vi "Path_Test_2020_TankRobot_Ramsete_ScanIndex_CreateFile.vi"() -> ()   [LabVIEW 2019]
uses:
  Pathfinder-Lib/VIs/Waypoint.ctl
  <vilib>/Rock Robotics/WPI/DriverStation/WPI_DriverStationRobotMode2.ctl
  Pathfinder-Lib/VIs/Wheel_Ctrl_Path_Element.ctl
  PathExecution_Library/PATH_SAMPLE.ctl
  PathExecution_Library/POSE.ctl
  PathExecution_Library/TRANSLATION.ctl
  PathExecution_Library/ROTATION.ctl
  Pathfinder-Lib/VIs/Wheel_Ctrl_Path.ctl
  <vilib>/Rock Robotics/SystemInterfaces/AI/FPGA_AIGyroChannel.ctl
  <vilib>/Rock Robotics/SystemInterfaces/DIO/FPGA_DIOChannel.ctl
  <vilib>/Rock Robotics/WPI/Encoder/WPI_EncoderType.ctl
  <vilib>/Rock Robotics/SystemInterfaces/DIO/FPGA_DIOPWMChannel.ctl
  <vilib>/Rock Robotics/WPI/SafetyOutput/WPI_SafetyOutputConfigMenu.ctl
  <vilib>/Rock Robotics/WPI/Gyro/WPI_GyroAnalogOpen.vi
  <vilib>/Rock Robotics/WPI/Counter/WPI_CounterDigitalInputToDigitalSource.vi
  <vilib>/Rock Robotics/WPI/RobotDrive/WPI_RobotDriveOpen2MotorWithTalon.vi
  Robot Global Data.vi
  <vilib>/Rock Robotics/Network Tables/NT Write Numeric Array.vi
  <vilib>/addons/control/pid/pid.llb/PID (DBL).vi
  <vilib>/Rock Robotics/Network Tables/NT Write Number.vi
  Pathfinder-Lib/Pathfinder.lvlib
  Secret_Control_Library_Protected/Secret_Control_Library_Protected.lvlib
  PathExecution_Library/PathExecution_Library.lvlib
  <vilib>/addons/control/pid/NI_PID_pid.lvlib
panel:
  in  "Tab Control 3":enum32{"Robot Data", "Path Definition"}(tab)
  in  "Real max\n speed":dbl=96.0
  in  "wheelbase_width":dbl=20.866
  in  "max_jerk":dbl=90.0
  in  "max_acceleration":dbl=65.0
  in  "max_velocity":dbl=72.0
  in  "?":T1[](array[typedef])=[{"x"=15.0, "y"=105.0, "angle"=0.0}, {"x"=35.0, "y"=105.0, "angle"=0.0}, {"x"=210.0, "y"=185.0, "angle"=60.0}]
  in  "Path Results\ndT":dbl=0.02 format="%7.3f"
  in  "sample_count":i32=100000
  out "Path calculation error":errorcluster
  in  "Calculate\nPath":bool
  out "Complete,\nReady to \nExecute":bool
  out "Path \nSpeed > \nMax":bool
  in  "Rev\nDirection":bool
  out "max speed":dbl
  in  "Tab Control 2":T2(tab)
  out "Robot Mode":T3
  in  "Enable Ramsete":bool=TRUE
  out "Distance":dbl[](array[numeric]) format="%19.2f"
  out "Heading":dbl format="%18.2f"
  in  "Execute\nRobot":bool
  out "Robot\nExecuting":bool
  in  "Stop\nProgram":bool
  out "DistRead":dbl[](array[numeric]) format="%19.2f"
  out "Speed":dbl[](array[numeric]) format="%19.2f"
  in  "Speed PID":T4={"proportional gain (Kc)"=0.5, "integral time (Ti, min)"=0.015, "derivative time (Td, min)"=0.0} {"derivative time (Td, min)" format="%.3f"; "integral time (Ti, min)" format="%.3f"; "proportional gain (Kc)" format="%.3f"}
  out "SpeedDmd":dbl[](array[numeric]) format="%19.2f"
  out "MotorOut":dbl[](array[numeric]) format="%19.2f"
  in  "Include Step":bool=TRUE
  in  "End Path CMD":i32=64
  in  "Cont Path CMD":i32=62
  in  "Start Path CMD":i32=60
  in  "Starting Step":i32
  in  "Command List Path Comment":string
  in  "Command List File Name":path
  in  "CreateCmdList":bool
  in  "CreateCmdList 2":bool
  in  "Command List File Name 2":path
  in  "Command List Path Comment 2":string
  in  "Starting Step 2":i32
  in  "Start Path CMD 2":i32=80
  in  "Cont Path CMD 2":i32=82
  in  "End Path CMD 2":i32=84
  in  "Include Step 2":bool=TRUE
  in  "Tab Control":T5(tab)
  out "Position":cluster{dbl[], dbl[]}[](graph)
  out "Path":T6(graph)
  out "Size":i32
  out "Robot Path Data":T7[](array[typedef]) {"D Time" format="%13.3f"; "Angle" format="%13.3f"; "R dist" format="%13.3f"; "L dist" format="%13.3f"; "R spd" format="%13.3f"; "L spd" format="%13.3f"; "T Time" format="%13.3f"}
  out "Ramsete Path":T8[](array[typedef])
  out "element":T8
  out "AtReference":bool
  out "size(s)":i32
  out "Path INX":i32
  out "size(s) 2":i32
  out "Err Pose":T9
  out "CurrentRelativePose":T9
  out "Des Pose":T9
  # "ROBOT DATA"
  # "INCHES/SEC"
  # "INCHES/SEC"
  # "INCHES/SEC^2"
  # "?? INCHES/SEC^3"
  # "Simulated robot is 20.866"
  # "INCHES"
  # "PATH DEFINITION"
  # "SEC"
  # "ROBOT EXECUTION"
  # "Instructions:\nThis should create a path, show the data on the various tabs and optionally write the motor demands and expected results to a file for use on a a robot..\n1) Enter robot data on Robot Data Tab\n2) Define your path definitions.\n3) Define the time increment.  0.020 is chosen since that matches the normal loop time.\n4) Press calculate path.  If a good path was calculated it will be displayed on the Tank Data tab, and the Ready to Execute will indicate execution can begin.\nThe path can be recalculated many times before selecting execute.\n\nTo write to a file.\n5) Select the file name\n6) This example uses \"steps\", sequential numbers for inclusion into a list based autonomous routine.  Including the step number if optional.\n7) This uses command numbers to indicate first, last, and intermediate steps.  This allows some simplification of the execution routine.  It\nalso allows the path to be executed backwards if desired.  The command numbers are changeable.\n8) Press \"Create Command List\".\n\nNotes:\n- PC robot simulataion is disabled in this program.  The code is still there if you want to restore it and try it out.  Use one of the other test programs \nto simulate the path on a PC.\n- The path generation logic doesn't account distribution of speed to the left and right wheels.  As a result the maximum speed can be exceeded.\nIf this happens, but Path Speed > Max light will light and Ready to Execute will not light.  Lower the maximum speed in the Robot Data tab\nand recalulate the path.\n- 2019 playing field size - width: 26 ft 11.25 In = 323.25 in , length: 52 ft 5.25 in = 629.25 in  (I didn't verify this for the 2020 version.)"
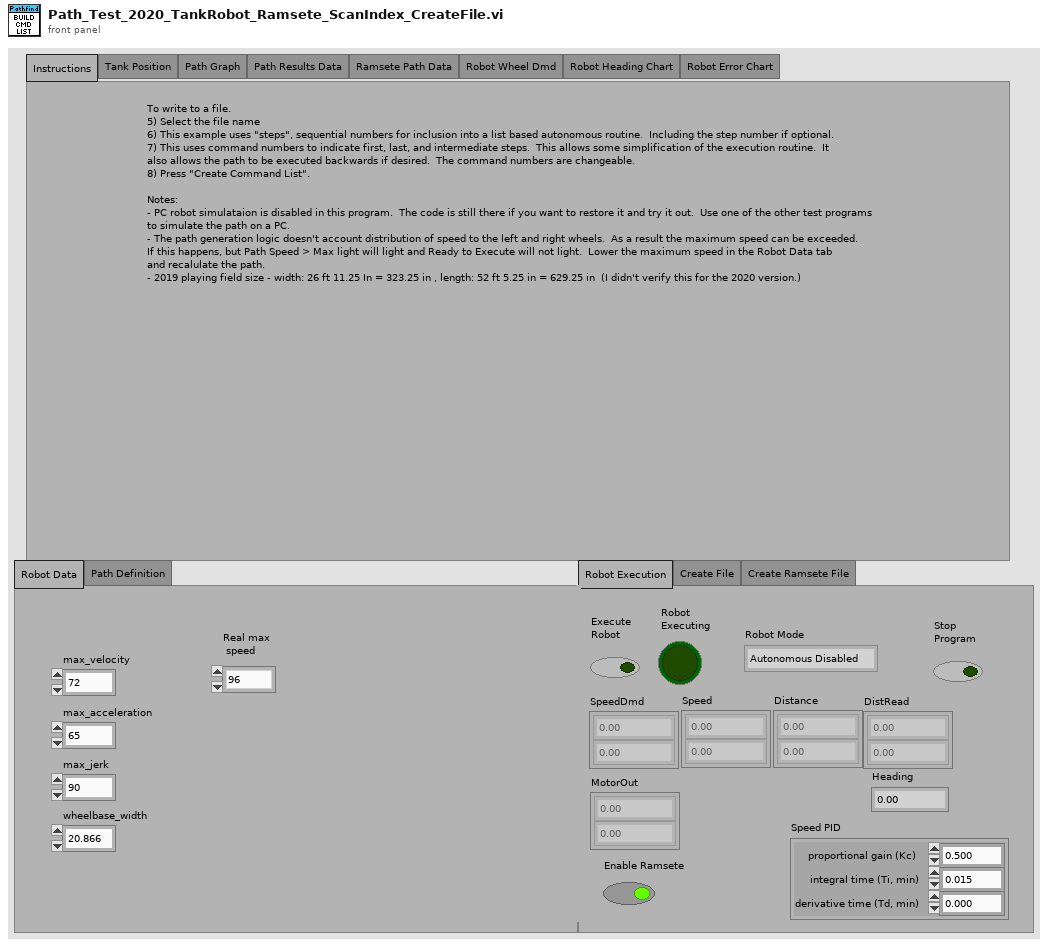
[diagram p1: front panel]
types:
  T1 = typedef "Pathfinder.lvlib/Waypoint.ctl" = cluster{"x":dbl, "y":dbl, "angle":dbl}
  T2 = enum32{"Robot Execution", "Create File", "Create Ramsete File"}
  T3 = typedef "WPI_DriverStationRobotMode2.ctl" = enum16{"Autonomous Disabled", "Autonomous Enabled", "Teleop Disabled", "Teleop Enabled", "Disconnected", "Finish", "Test Disabled", "Test Enabled", "Emergency Stopped"}
  T4 = cluster{"proportional gain (Kc)":dbl, "integral time (Ti, min)":dbl, "derivative time (Td, min)":dbl}
  T5 = enum32{"Instructions", "Tank Position", "Path Graph", "Path Results Data", "Ramsete Path Data", "Robot Wheel Dmd", "Robot Heading Chart", "Robot Error Chart"}
  T6 = cluster{"position":dbl, "velocity":dbl, "acceleration":dbl, "jerk":dbl, "heading":dbl}[]
  T7 = typedef "Pathfinder.lvlib/Wheel_Ctrl_Path_Element.ctl" = cluster{"T Time":dbl, "L spd":dbl, "R spd":dbl, "L dist":dbl, "R dist":dbl, "Angle":dbl, "D Time":dbl}
  T8 = typedef "PathExecution_Library.lvlib/PATH_SAMPLE.ctl" = cluster{"Path Lin Vel":dbl, "Path Ang Vel":dbl, "Path X":dbl, "Path Y":dbl, "Path Heading":dbl, "Path Time Off":dbl}
  T9 = typedef "PathExecution_Library.lvlib/POSE.ctl" = cluster{"TRANSLATION":T10, "ROTATION":T11}
  T10 = typedef "PathExecution_Library.lvlib/TRANSLATION.ctl" = cluster{"X":dbl, "Y":dbl}
  T11 = typedef "PathExecution_Library.lvlib/ROTATION.ctl" = cluster{"VALUE":dbl, "COS":dbl, "SIN":dbl}
  T12 = typedef "Pathfinder.lvlib/Wheel_Ctrl_Path.ctl" = cluster{"Wheel_Ctrl_Elements":T7[], "NumberOfElements":u32, "DeltaMillseconds":i32}
  T13 = typedef "Pathfinder.lvlib/Segment.ctl" = cluster{"dt":dbl, "x":dbl, "y":dbl, "position":dbl, "velocity":dbl, "acceleration":dbl, "jerk":dbl, "heading":dbl}
  T14 = cluster{"position":dbl, "velocity":dbl, "acceleration":dbl, "jerk":dbl, "heading":dbl}
  T15 = typedef "PathExecution_Library.lvlib/CHASSIS.ctl" = cluster{"vX":dbl, "vY":dbl, "vOmega":dbl}
  T16 = typedef "WPI_SafetyOutputConfigMenu.ctl" = enum16{"Enable", "Disable"}
  T17 = typedef "WPI_EncoderType.ctl" = enum16{"1x", "2x", "4x"}
  T18 = typedef "FPGA_AIGyroChannel.ctl" = enum8{"AI 0", "AI 1", "Invalid"}
  T19 = typedef "FPGA_DIOPWMChannel.ctl" = enum8{"PWM 0", "PWM 1", "PWM 2", "PWM 3", "PWM 4", "PWM 5", "PWM 6", "PWM 7", "PWM 8", "PWM 9", "PWM MXP 0", "PWM MXP 1", "PWM MXP 2", "PWM MXP 3", "PWM MXP 4", "PWM MXP 5", "PWM MXP 6", "PWM MXP 7", "PWM MXP 8", "PWM MXP 9", "Invalid"}
  T20 = typedef "FPGA_DIOChannel.ctl" = enum8{"DIO 0", "DIO 1", "DIO 2", "DIO 3", "DIO 4", "DIO 5", "DIO 6", "DIO 7", "DIO 8", "DIO 9", "DIO MXP 0", "DIO MXP 1", "DIO MXP 2", "DIO MXP 3", "DIO MXP 4", "DIO MXP 5", "DIO MXP 6", "DIO MXP 7", "DIO MXP 8", "DIO MXP 9", "DIO MXP 10", "DIO MXP 11", "DIO MXP 12", "DIO MXP 13", "DIO MXP 14", "DIO MXP 15", "SPI Port CS1", "SPI Port CS2", "SPI Port CS3", "SPI Port MISO", "SPI Port MOSI", "Invalid"}
  T21 = typedef "WPI_RobotDriveDevRef.ctl" = cluster{"DevStatus":errorcluster, "Motors[]":T22[], "Square Inputs":bool, "Max Output":dbl}
  T22 = typedef "WPI_MotorControlDeviceRef.ctl" = cluster{"DeviceStatus":errorcluster, "Type":T23, "PWM":cluster{"PWM Channel":T19, "DeadBand":T24}, "CAN":cluster{"Device Number":u8, "SetOutput VI Ref":variant, "GetOutput VI Ref":variant, "Enable VI Ref":variant, "Disable VI Ref":variant, "Data":variant}, "Invert":bool, "DIO PWM":cluster{"PWM \"Enable\" Channel":T19, "DIOChannel":T20, "PWM Rate":dbl}}
  T23 = typedef "WPI_MotorControlType.ctl" = enum16{"PWM", "CAN", "DIO PWM"}
  T24 = typedef "WPI_PWMDeadband.ctl" = cluster{"Name":string, "maxPositivePwm":i32, "minPositivePwm":i32, "centerPwm":i32, "maxNegativePwm":i32, "minNegativePwm":i32, "angularRange":u16}
  T25 = typedef "WPI_DigitalInputDevRef.ctl" = cluster{"DevStatus":errorcluster, "DIO Channel":T20}
  T26 = typedef "FPGA_CounterEncoderSourceConvertionLVSourceType.ctl" = cluster{"DevStatus":errorcluster, "AnalogTriggerMode?":bool, "DigitalMode":cluster{"DIO Channel":T27}, "AnalogTriggerMode":cluster{"AnalogTriggerIndex":T28, "OutputType":T29}}
  T27 = typedef "FPGA_DIODigitalSourceChannel.ctl" = enum8{"DIO 0", "DIO 1", "DIO 2", "DIO 3", "DIO 4", "DIO 5", "DIO 6", "DIO 7", "DIO 8", "DIO 9", "DIO MXP 0", "DIO MXP 1", "DIO MXP 2", "DIO MXP 3", "DIO MXP 4", "DIO MXP 5", "DIO MXP 6", "DIO MXP 7", "DIO MXP 8", "DIO MXP 9", "DIO MXP 10", "DIO MXP 11", "DIO MXP 12", "DIO MXP 13", "DIO MXP 14", "DIO MXP 15", "SPI Port CS1", "SPI Port CS2", "SPI Port CS3", "SPI Port MISO", "SPI Port MOSI", "Disabled"}
  T28 = typedef "FPGA_AnalogTriggerIndex.ctl" = enum8{"Trig 0", "Trig 1", "Trig 2", "Trig 3", "Trig 4", "Trig 5", "Trig 6", "Trig 7", "Invalid"}
  T29 = typedef "FPGA_AnalogTriggerOutType.ctl" = enum16{"InWindow", "TriggerState", "Rising", "Falling"}
  T30 = typedef "WPI_EncoderDevRef.ctl" = cluster{"DevStatus":errorcluster, "EncoderIndex":T31, "CounterIndex":T32, "DistancePerCount":dbl, "Decoding Type":T17}
  T31 = typedef "FPGA_EncoderIdx.ctl" = enum8{"Enc 0", "Enc 1", "Enc 2", "Enc 3", "Enc 4", "Enc 5", "Enc 6", "Enc 7", "Invalid"}
  T32 = typedef "FPGA_CounterCtrSystemIndex.ctl" = enum8{"Ctr 0", "Ctr 1", "Ctr 2", "Ctr 3", "Ctr 4", "Ctr 5", "Ctr 6", "Ctr 7", "Invalid"}
  T33 = typedef "WPI_GyroDevRef.ctl" = cluster{"DevStatus":errorcluster, "Analog Channel":T34, "Gain (VoltsPerDegree/Second)":dbl, "Gyro Type":enum16{"Analog", "XRS450"}, "Handle":i32, "SPI Bus":T35, "Device Found":bool, "Sample Rate":dbl, "Calibrate On Open":bool, "Offset":dbl}
  T34 = typedef "FPGA_AIChannel.ctl" = enum8{"AI 0", "AI 1", "AI 2", "AI 3", "AI MXP 0", "AI MXP 1", "AI MXP 2", "AI MXP 3", "Invalid"}
  T35 = typedef "spi_bus.ctl" = enum16{"SPI On-Board, CS0", "SPI On-Board, CS1", "SPI On-Board, CS2", "SPI On-Board, CS3", "SPI MXP", "Invalid"}
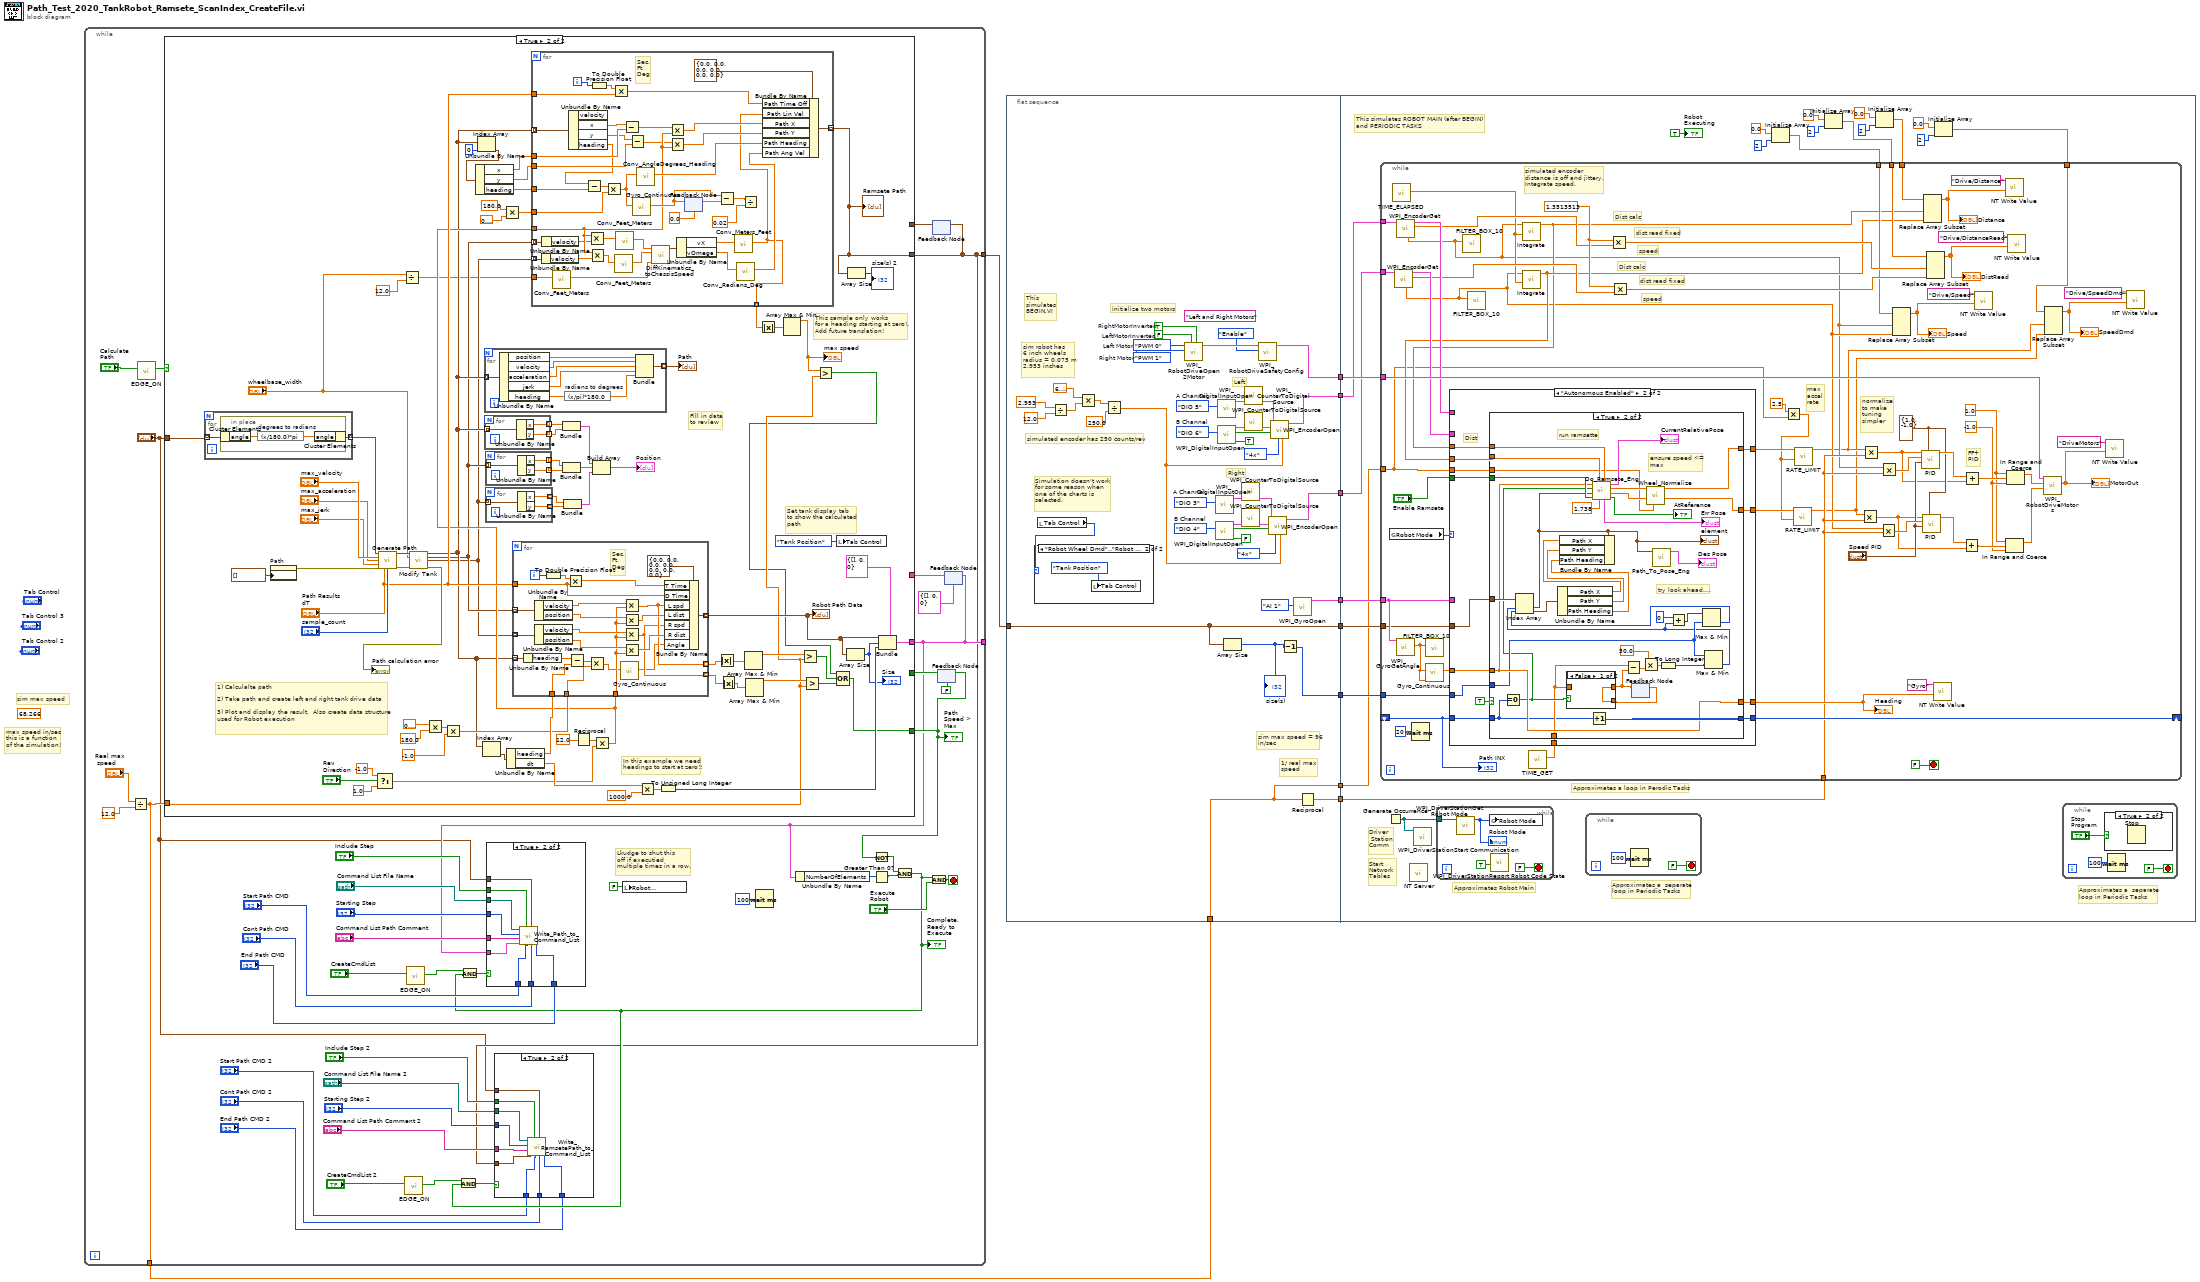
[diagram p0: block diagram]
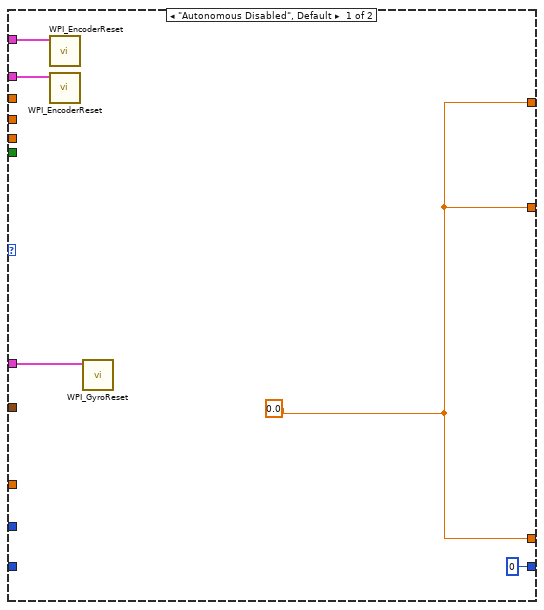
[diagram p4: hidden frame]
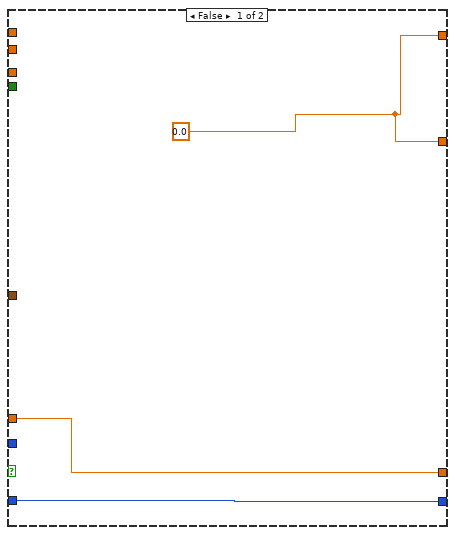
[diagram p5: hidden frame]
diagram:
  (unwired) 68.266 ("x")
  # "sim max speed"
  # "max speed in/sec\nthis is a function\nof the simulation!"
  n1 = while {
    tunnel: [w26] -> w10
    tunnel: [w25] -> _
    tunnel: [w12] -> w4
    stop <- w45 stop-if-true
    # "Lkudge to shut this\noff if executied\nmultiple times in a row."
    n2 = Divide(x="Real max\n speed", y=12.0) -> (x/y=w26:dbl)
    n3 = call "EDGE_ON.vi"("INPUT"="Calculate\nPath") -> ("EDGE ON"=w50:bool)  [unwired: 10 in]
    n4 = call "EDGE_ON.vi"("INPUT"="CreateCmdList 2") -> ("EDGE ON"=w19:bool)  [unwired: 10 in]
    n5 = call "EDGE_ON.vi"("INPUT"="CreateCmdList") -> ("EDGE ON"=w33:bool)  [unwired: 10 in]
    n6 = local write "Robot\nExecuting"(FALSE ("Robot\nExecuting")) -> ()
    n7 = Wait (ms)(milliseconds to wait=u32 100) -> ()  [unwired: 1 out]
    n8 = feedback #1() -> (w24:T8[])  [unwired: 1 in]
    n9 = feedback #2(FALSE) -> (w42:bool)
    n10 = feedback #3(T12 {"Wheel_Ctrl_Elements"=[], "NumberOfElements"=0, "DeltaMillseconds"=0} ("Wheel_Ctrl_Elements")) -> (w48:T12)
    n11 = case shown="True" w50 {
      tunnel: [w73 w117] -> w25
      tunnel: w48 -> [w73 _]
      tunnel: w26 -> [_ w76]
      tunnel: [w72 w114] -> w39
      tunnel: w42 -> [w72 _]
      tunnel: "?" -> [_ w112]
      tunnel: [w71 w96] -> w12
      tunnel: w24 -> [w71 _]
      frame False {
      }
      frame True {
        # "This sample only works\nfor a heading starting at zero!.\nAdd future translation!"
        # "Set tank display tab\nto show the calculated\npath"
        # "Fill in data\nto review"
        # "1) Calculalte path\n\n2) Take path and create left and right tank drive data\n\n3) Plot and display the result.  Also create data structure\nused for Robot execution"
        # "In this example we need\nheadings to start at zero!!"
        n12 = for {
          tunnel: w112 -> [w217] mode=indexing
          tunnel: [w216] -> w142 mode=indexing
          n13 = in-place {
            n14 = in-place-cluster #4(w217) -> ("angle"=w219:dbl)
            n15 = expression code="(x/180.0)*pi" "degrees to radians"(w219) -> (w218:dbl)
            n16 = in-place-cluster #4("angle"=w218) -> (w216:T1)
          }
        }
        n17 = property on="Path" class="WFChart (strict)"("History Data"=T6 []) -> (error out=w143:errorcluster)  [unwired: 2 in, 1 out]
        n18 = Select(t=-1.0, s="Rev\nDirection", f=1.0) -> (s? t:f=w107:dbl)
        n19 = call "Generate Path.vi"("path"=w142, "max_velocity"="max_velocity", "max_acceleration"="max_acceleration", "max_jerk"="max_jerk", "error in"=w143, "dt (.001)"="Path Results\ndT", "sample_count (100000)"="sample_count") -> ("Segments"=w144:T13[], "error out"=w132:errorcluster)  [unwired: 7 in]
        n20 = Divide(x="wheelbase_width", y=12.0) -> (x/y=w86:dbl)
        n21 = call "Modify Tank.vi"("Original"=w144, "wheelbase_width"="wheelbase_width", "error in"=w132) -> ("original"=w101:T13[], "left"=w90:T13[], "right"=w89:T13[], "error out"=→"Path calculation error":errorcluster)  [unwired: 9 in]
        n22 = Multiply(x=0.3183098861837907, y=180.0) -> (x*y=w148:dbl)
        n23 = Multiply(x=w148, y=-1.0) -> (x*y=w104:dbl)
        n24 = Index Array(array=w101, index=0) -> (element=w99:T13)
        n25 = Unbundle By Name(w99) -> ("x"=w98:dbl, "y"=w97:dbl, "heading"=w94:dbl)
        n26 = Index Array(array=w101) -> (element=w149:T13)  [unwired: 1 in]
        n27 = for {
          tunnel: w101 -> [w236] mode=indexing
          tunnel: [w230] -> w146 mode=indexing
          n28 = Unbundle By Name(w236) -> ("position"=w235:dbl, "velocity"=w234:dbl, "acceleration"=w233:dbl, "jerk"=w232:dbl, "heading"=w231:dbl)
          n29 = expression code="(x/pi)*180.0" "radians to degrees"(w231) -> (w229:dbl)
          n30 = Bundle("position"=w235, "velocity"=w234, "acceleration"=w233, "jerk"=w232, "heading"=w229) -> (w230:T14)  [unwired: 1 in]
        }
        "Path" <- w146
        n31 = for {
          tunnel: w101 -> [w222] mode=indexing
          tunnel: [w221] -> w139 mode=indexing
          tunnel: [w220] -> w140 mode=indexing
          n32 = Unbundle By Name(w222) -> ("x"=w221:dbl, "y"=w220:dbl)
        }
        n33 = for {
          tunnel: w90 -> [w228] mode=indexing
          tunnel: [w227] -> w133 mode=indexing
          tunnel: [w226] -> w134 mode=indexing
          n34 = Unbundle By Name(w228) -> ("x"=w227:dbl, "y"=w226:dbl)
        }
        n35 = for {
          tunnel: w89 -> [w225] mode=indexing
          tunnel: [w224] -> w135 mode=indexing
          tunnel: [w223] -> w136 mode=indexing
          n36 = Unbundle By Name(w225) -> ("x"=w224:dbl, "y"=w223:dbl)
        }
        n37 = Multiply(x=180.0, y=0.3183098861837907) -> (x*y=w91:dbl)
        n38 = Unbundle By Name(w149) -> ("heading"=w105:dbl, "dt"=w121:dbl)
        n39 = Bundle(w139, w140) -> (w141:cluster{dbl[], dbl[]})  [unwired: 1 in]
        n40 = Bundle(w133, w134) -> (w138:cluster{dbl[], dbl[]})  [unwired: 1 in]
        n41 = Bundle(w135, w136) -> (w137:cluster{dbl[], dbl[]})  [unwired: 1 in]
        n42 = Reciprocal(x=12.0) -> (1/x=w111:dbl)
        n43 = Build Array(w141, w138, w137) -> (→"Position":cluster{dbl[], dbl[]}[])
        n44 = Multiply(x=w111, y=w107) -> (x*y=w103:dbl)
        n45 = for {
          tunnel: "Path Results\ndT" -> [w211]
          tunnel: [w214] -> w113 mode=indexing
          tunnel: w103 -> [w206]
          tunnel: w90 -> [w203] mode=indexing
          tunnel: w89 -> [w202] mode=indexing
          tunnel: w101 -> [w201] mode=indexing
          tunnel: w105 -> [w194]
          tunnel: [w197] -> w85 mode=indexing
          tunnel: [w196] -> w82 mode=indexing
          tunnel: w104 -> [w195]
          i -> [w213]
          # "Sec,\nFt,\nDeg"
          n46 = Unbundle By Name(w201) -> ("heading"=w199:dbl)
          n47 = Unbundle By Name(w203) -> ("velocity"=w210:dbl, "position"=w209:dbl)
          n48 = Unbundle By Name(w202) -> ("velocity"=w208:dbl, "position"=w207:dbl)
          n49 = To Double Precision Float(number=w213) -> (double precision float=w215:dbl)
          n50 = Multiply(x=w215, y=w211) -> (x*y=w212:dbl)
          n51 = Subtract(x=w199, y=w194) -> (x-y=w200:dbl)
          n52 = Multiply(x=w200, y=w195) -> (x*y=w193:dbl)
          n53 = call "Gyro_Continuous.vi"("GyroInput"=w193) -> ("GyroContinuous"=w192:dbl)  [unwired: 10 in]
          n54 = Multiply(x=w210, y=w206) -> (x*y=w197:dbl)
          n55 = Multiply(x=w209, y=w206) -> (x*y=w205:dbl)
          n56 = Multiply(x=w208, y=w206) -> (x*y=w196:dbl)
          n57 = Multiply(x=w207, y=w206) -> (x*y=w204:dbl)
          n58 = Bundle By Name(cluster=T7 {"T Time"=0.0, "L spd"=0.0, "R spd"=0.0, "L dist"=0.0, "R dist"=0.0, "Angle"=0.0, "D Time"=0.0} ("Wheel dmd"), "T Time"=w212, "D Time"=w211, "L spd"=w197, "L dist"=w205, "R spd"=w196, "R dist"=w204, "Angle"=w192) -> (w214:T7)
        }
        "Robot Path Data" <- w113
        n59 = for {
          tunnel: "Path Results\ndT" -> [w189]
          tunnel: w103 -> [w164]
          tunnel: w101 -> [w188] mode=indexing
          tunnel: [w182] -> w96 mode=indexing
          tunnel: w98 -> [w175]
          tunnel: w97 -> [w173]
          tunnel: w94 -> [w170]
          tunnel: w91 -> [w167]
          tunnel: w90 -> [w166] mode=indexing
          tunnel: w89 -> [w165] mode=indexing
          tunnel: w86 -> [w161]
          tunnel: [w151] -> w77 mode=indexing
          i -> [w190]
          # "Sec,\nFt,\nDeg"
          n60 = Unbundle By Name(w165) -> ("velocity"=w162:dbl)
          n61 = Unbundle By Name(w166) -> ("velocity"=w163:dbl)
          n62 = call "Conv_Feet_Meters.vi"("Feet"=w161) -> ("Meters"=w156:dbl)  [unwired: 10 in]
          n63 = Unbundle By Name(w188) -> ("x"=w176:dbl, "y"=w174:dbl, "heading"=w171:dbl)  [unwired: 1 out]
          n64 = Subtract(x=w171, y=w170) -> (x-y=w186:dbl)
          n65 = Multiply(x=w164, y=w163) -> (x*y=w160:dbl)
          n66 = Multiply(x=w164, y=w162) -> (x*y=w159:dbl)
          n67 = To Double Precision Float(number=w190) -> (double precision float=w191:dbl)
          n68 = Multiply(x=w186, y=w167) -> (x*y=w169:dbl)
          n69 = Multiply(x=w191, y=w189) -> (x*y=w185:dbl)
          n70 = call "Conv_Feet_Meters.vi"("Feet"=w159) -> ("Meters"=w157:dbl)  [unwired: 10 in]
          n71 = call "Conv_Feet_Meters.vi"("Feet"=w160) -> ("Meters"=w158:dbl)  [unwired: 10 in]
          n72 = Subtract(x=w176, y=w175) -> (x-y=w172:dbl)
          n73 = Subtract(x=w174, y=w173) -> (x-y=w150:dbl)
          n74 = call "Gyro_Continuous.vi"("GyroInput"=w169) -> ("GyroContinuous"=w177:dbl)  [unwired: 10 in]
          n75 = call "Conv_AngleDegrees_Heading.vi"("Degrees"=w169) -> ("Radians"=w168:dbl)  [unwired: 10 in]
          n76 = call "DiffKinematics_toChassisSpeed.vi"("TrackWidth_Meters"=w156, "RightVelocity"=w157, "LeftVelocity"=w158) -> ("CHASSIS Speed"=w155:T15)  [unwired: 8 in]
          n77 = Multiply(x=w172, y=w164) -> (x*y=w184:dbl)
          n78 = Multiply(x=w150, y=w164) -> (x*y=w183:dbl)
          n79 = Unbundle By Name(w155) -> ("vX"=w154:dbl, "vOmega"=w153:dbl)
          n80 = feedback-in #5(w177) -> ()
          n81 = feedback #5(0.0) -> (w180:dbl)
          n82 = Subtract(x=w177, y=w180) -> (x-y=w179:dbl)
          n83 = call "Conv_Meters_Feet.vi"("Meters"=w154) -> ("Feet"=w151:dbl)  [unwired: 10 in]
          n84 = call "Conv_Radians_Deg.vi"("Radians"=w153) -> ("Degrees"=w152:dbl)  [unwired: 10 in]
          n85 = Divide(x=w179, y=0.02) -> ()  [unwired: 1 out]
          n86 = Bundle By Name(cluster=T8 {"Path Lin Vel"=0.0, "Path Ang Vel"=0.0, "Path X"=0.0, "Path Y"=0.0, "Path Heading"=0.0, "Path Time Off"=0.0} ("Path Sample"), "Path Time Off"=w185, "Path Lin Vel"=w151, "Path X"=w184, "Path Y"=w183, "Path Heading"=w168, "Path Ang Vel"=w152) -> (w182:T8)
        }
        "Ramsete Path" <- w96
        n87 = Multiply(x=w121, y=1000.0) -> (x*y=w119:dbl)
        n88 = To Unsigned Long Integer(number=w119) -> (unsigned 32bit integer=w118:u32)
        n89 = Absolute Value(x=w85) -> (abs(x)=w84:dbl[])
        n90 = Absolute Value(x=w82) -> (abs(x)=w80:dbl[])
        n91 = Array Max & Min(array=w84) -> (max value=w83:dbl)  [unwired: 3 out]
        n92 = Array Max & Min(array=w80) -> (max value=w81:dbl)  [unwired: 3 out]
        n93 = Absolute Value(x=w77) -> (abs(x)=w78:dbl[])
        n94 = Array Max & Min(array=w78) -> (max value=w75:dbl)  [unwired: 3 out]
        "max speed" <- w75
        n95 = Greater?(x=w83, y=w76) -> (0:w115:bool)
        n96 = Greater?(x=w81, y=w76) -> (0:w79:bool)
        n97 = Greater?(x=w75, y=w76) -> (0:w74:bool)
        n98 = Compound Arithmetic op=OR(w74, w115, w79) -> (w114:bool)
        n99 = local write "Tab Control"(T5."Tank Position" ("Tab Control")) -> ()
        n100 = Array Size(array=w113) -> (size(s)=w116:i32)
        "Size" <- w116
        n101 = Array Size(array=w96) -> (size(s)=→"size(s) 2":i32)
        n102 = Bundle(cluster=T12 {"Wheel_Ctrl_Elements"=[], "NumberOfElements"=0, "DeltaMillseconds"=0} ("Wheel_Ctrl_Elements"), "Wheel_Ctrl_Elements"=w113, "NumberOfElements"=w116, "DeltaMillseconds"=w118) -> (w117:T12)
      }
    }
    "Path \nSpeed > \nMax" <- w39
    n103 = Unbundle By Name(w25) -> ("NumberOfElements"=w47:u32)
    n104 = Not(x=w39) -> (.not. x?=w40:bool)
    n105 = Greater Than 0?(x=w47) -> (x > 0?=w41:bool)
    n106 = And(x=w40, y=w41) -> (x .and. y?=w17:bool)
    "Complete,\nReady to \nExecute" <- w17
    n107 = And(x=w19, y=w17) -> (x .and. y?=w18:bool)
    n108 = And(x=w33, y=w17) -> (x .and. y?=w34:bool)
    n109 = case shown="True" w34 {
      tunnel: "Command List File Name" -> [_ w70]
      tunnel: "Starting Step" -> [_ w69]
      tunnel: "Command List Path Comment" -> [_ w68]
      tunnel: w25 -> [_ w67]
      tunnel: "End Path CMD" -> [_ w66]
      tunnel: "Cont Path CMD" -> [_ w65]
      tunnel: "Start Path CMD" -> [_ w64]
      tunnel: "Include Step" -> [_ w63]
      tunnel: "?" -> [_ w62]
      frame False {
      }
      frame True {
        n110 = call "Write_Path_to_Command_List.vi"("LastCmdNumb"=w66, "CmdNumb"=w65, "WayPoints"=w62, "FirstCmdNumb"=w64, "Include Step"=w63, "Wheel_Ctrl_Elements"=w67, "Comment"=w68, "starting step"=w69, "Cmd List File"=w70) -> ()  [unwired: 3 in]
      }
    }
    n111 = case shown="True" w18 {
      tunnel: "Command List File Name 2" -> [_ w61]
      tunnel: "Starting Step 2" -> [_ w60]
      tunnel: "Command List Path Comment 2" -> [_ w59]
      tunnel: w12 -> [_ w53]
      tunnel: "End Path CMD 2" -> [_ w58]
      tunnel: "Cont Path CMD 2" -> [_ w57]
      tunnel: "Start Path CMD 2" -> [_ w56]
      tunnel: "Include Step 2" -> [_ w55]
      tunnel: "?" -> [_ w54]
      frame False {
      }
      frame True {
        n112 = call "Write_RamsetePath_to_Command_List.vi"("LastCmdNumb"=w58, "CmdNumb"=w57, "WayPoints"=w54, "FirstCmdNumb"=w56, "Include Step"=w55, "Path Sample Array"=w53, "Comment"=w59, "starting step"=w60, "Cmd List File"=w61) -> ()  [unwired: 3 in]
      }
    }
    n113 = And(x=w17, y="Execute\nRobot") -> (x .and. y?=w45:bool)
    n114 = feedback-in #1(w12) -> ()
    n115 = feedback-in #2(w39) -> ()
    n116 = feedback-in #3(w25) -> ()
  }
  n117 = flat-sequence {
    tunnel: [w252] -> w9
    tunnel: [w275] -> w8
    tunnel: [w250] -> w7
    tunnel: [w251] -> w6
    tunnel: [w249] -> w5
    tunnel: w10 -> [w237]
    tunnel: w4 -> [w247]
    tunnel: [w247] -> w3
    tunnel: [w245] -> w2
    tunnel: [w237] -> w1
    tunnel: w9 -> [w298]
    tunnel: w8 -> [w297]
    tunnel: w7 -> [w296]
    tunnel: w6 -> [w293]
    tunnel: w5 -> [w284]
    tunnel: w3 -> [w291]
    tunnel: w2 -> [w290]
    tunnel: w1 -> [w278]
    frame #0 {
      w262 = FPGA_DIOPWMChannel."PWM 1"  # Right Motor
      w261 = FPGA_DIOPWMChannel."PWM 0"  # Left Motor
      (unwired) "Left and Right Motors" ("refnum name")
      w263 = FALSE  # LeftMotorInverted
      w264 = TRUE  # RightMotorInverted
      w260 = FPGA_DIOChannel."DIO 4"  # B Channel
      w259 = FPGA_DIOChannel."DIO 3"  # A Channel
      w256 = FPGA_DIOChannel."DIO 6"  # B Channel
      w255 = FPGA_DIOChannel."DIO 5"  # A Channel
      # "sim max speed = 96\nin/sec"
      # "1/ real max \nspeed"
      # "simulated encoder has 250 counts/rev"
      # "Simulation doesn't work\nfor some reason when\none of the charts is\nselected."
      # "This \nsimulates\nBEGIN.VI"
      # "sim robot has\n6 inch wheels\nradius = 0.075 m\n2.953 inches"
      # "initialize two motors"
      # "Right"
      # "Left"
      n118 = local read "Tab Control"() -> (w248:T5)
      n119 = case shown="\"Robot Wheel Dmd\"..\"Robot Error Chart\"" w248 {
        frame Default {
        }
        frame "Robot Wheel Dmd".."Robot Error Chart" {
          n120 = local write "Tab Control"(T5."Tank Position" ("Tab Control")) -> ()
        }
      }
      n121 = Divide(x=2.953, y=12.0) -> (x/y=w243:dbl)
      n122 = Multiply(x=6.283185307179586, y=w243) -> (x*y=w244:dbl)
      n123 = Divide(x=w244, y=250.0) -> (x/y=w238:dbl)
      n124 = call-poly <vilib>:"WPI_RobotDriveOpen2Motor.vi"("Right Motor Inverted"=w264, "Left Motor Inverted"=w263, "Right Motor"=w262, "Left Motor"=w261) -> ("RobotDriveDevRef"=w274:T21)  [unwired: 1 in, 6 out]
      n125 = call <vilib>:"WPI_DigitalInputOpen.vi"("DIO Channel"=w259) -> ("DigitalInputDevRef"=w272:T25)  [unwired: 1 in, 9 out]
      n126 = call <vilib>:"WPI_DigitalInputOpen.vi"("DIO Channel"=w260) -> ("DigitalInputDevRef"=w271:T25)  [unwired: 1 in, 9 out]
      n127 = call <vilib>:"WPI_DigitalInputOpen.vi"("DIO Channel"=w255) -> ("DigitalInputDevRef"=w268:T25)  [unwired: 1 in, 9 out]
      n128 = call <vilib>:"WPI_DigitalInputOpen.vi"("DIO Channel"=w256) -> ("DigitalInputDevRef"=w267:T25)  [unwired: 1 in, 9 out]
      n129 = Array Size(array=w247) -> (size(s)=w246:i32)
      "size(s)" <- w246
      n130 = call-poly <vilib>:"WPI_CounterToDigitalSource.vi"("DigitalInputDevRef"=w272) -> ("Digital Source"=w273:T26)  [unwired: 6 out]
      n131 = call-poly <vilib>:"WPI_CounterToDigitalSource.vi"("DigitalInputDevRef"=w271) -> ("Digital Source"=w270:T26)  [unwired: 6 out]
      n132 = call-poly <vilib>:"WPI_CounterToDigitalSource.vi"("DigitalInputDevRef"=w268) -> ("Digital Source"=w269:T26)  [unwired: 6 out]
      n133 = call-poly <vilib>:"WPI_CounterToDigitalSource.vi"("DigitalInputDevRef"=w267) -> ("Digital Source"=w266:T26)  [unwired: 6 out]
      n134 = call <vilib>:"WPI_RobotDriveSafetyConfig.vi"("mode"=WPI_SafetyOutputConfigMenu."Enable", "RobotDriveDevRef"=w274) -> ("RobotDriveDevRef"=w252:T21)  [unwired: 8 in, 1 out]
      n135 = call <vilib>:"WPI_EncoderOpen.vi"("DistancePerCount"=w238, "Decoding Type"=WPI_EncoderType."4x", "Invert Direction (False)"=FALSE, "BSource"=w270, "ASource"=w273) -> ("EncoderDevRef"=w251:T30)  [unwired: 3 in, 3 out]
      n136 = call <vilib>:"WPI_EncoderOpen.vi"("DistancePerCount"=w238, "Decoding Type"=WPI_EncoderType."4x", "Invert Direction (False)"=TRUE, "BSource"=w266, "ASource"=w269) -> ("EncoderDevRef"=w250:T30)  [unwired: 3 in, 3 out]
      n137 = Decrement(x=w246) -> (x-1=w245:i32)
      n138 = call-poly <vilib>:"WPI_GyroOpen.vi"("Analog Channel"=FPGA_AIGyroChannel."AI 1") -> ("GyroDevRef"=w275:T33)  [unwired: 8 in, 2 out]
      n139 = Reciprocal(x=w237) -> (1/x=w249:dbl)
    }
    frame #1 {
      # "Approximates a  separate\nloop in Periodic Tasks"
      # "This simulates ROBOT MAIN (after BEGIN)\nand PERIODIC TASKS"
      # "Approximates a loop in Perodic Tasks"
      # "Approximates a  separate\nloop in Periodic Tasks"
      # "Approximates Robot Main"
      # "Start\nNetwork\nTables"
      # "Driver\n Station\nComm"
      n140 = Generate Occurrence() -> (w299:refnum<k4>)
      n141 = call <vilib>:"NT Server.vi"() -> ()  [unwired: 12 in]
      n142 = call <vilib>:"WPI_DriverStationStart Communication.vi"("occurrence"=w299) -> ()  [unwired: 11 in]
      n143 = while {
        tunnel: w299 -> [w432]
        stop <- FALSE stop-if-true
        n144 = call <vilib>:"WPI_DriverStationGet Robot Mode.vi"("DS Occurrence"=w432) -> ("Robot Mode"=w429:T3)  [unwired: 1 in, 9 out]
        "Robot Mode" <- w429
        n145 = global write "Robot Global Data.vi" "Robot Mode"(w429) -> ()
        n146 = call <vilib>:"WPI_DriverStationReport Robot Code State.vi"("TeleOp"=TRUE ("Autonomous")) -> ()  [unwired: 10 in, 1 out]
      }
      n147 = while {
        stop <- FALSE stop-if-true
        n148 = Wait (ms)(milliseconds to wait=u32 100) -> ()  [unwired: 1 out]
      }
      n149 = Initialize Array(0.0, 2 ("dimension size")) -> (w280:dbl[])
      n150 = Initialize Array(0.0, 2 ("dimension size")) -> (w281:dbl[])
      n151 = Initialize Array(0.0, 2 ("dimension size")) -> (w285:dbl[])
      n152 = Initialize Array(0.0, 2 ("dimension size")) -> (w279:dbl[])
      n153 = while {
        tunnel: w298 -> [w365]
        shift-right: [w364] -> _
        shift-left: _ -> [w348]
        tunnel: w297 -> [w361]
        tunnel: w296 -> [w360]
        tunnel: w280 -> [w337]
        tunnel: w293 -> [w352]
        tunnel: w291 -> [w350]
        tunnel: w290 -> [w349]
        tunnel: w281 -> [w338]
        tunnel: w285 -> [w339]
        tunnel: w284 -> [w322]
        tunnel: w279 -> [w315]
        tunnel: w278 -> [w305]
        stop <- FALSE stop-if-true
        w332 = -1.0 ("lower limit")
        w331 = 1.0 ("upper limit")
        w329 = cluster{"output high":dbl, "output low":dbl} {"output high"=1.0, "output low"=-1.0} ("output range")
        w343 = 1.3513513
        # "max\naccel\nrate"
        # "speed"
        # "dist read fixed"
        # "Dist calc"
        # "speed"
        # "dist read fixed"
        # "Dist calc"
        # "normalize\nto make\ntuning\nsimpler"
        # "FF+\nPID"
        # "simulated encoder\ndistance is off and jittery,\nIntegrate speed."
        n154 = global read "Robot Global Data.vi" "Robot Mode"() -> (w366:T3)
        n155 = call "TIME_ELAPSED.vi"() -> ("Elapsed Sec"=w320:dbl)  [unwired: 11 in]
        n156 = call <vilib>:"WPI_EncoderGet.vi"("EncoderDevRef"=w352) -> ("Distance"=w321:dbl, "EncoderDevRef"=w359:T30, "Rate"=w313:dbl)  [unwired: 5 in, 3 out]
        n157 = call <vilib>:"WPI_GyroGetAngle.vi"("GyroDevRef"=w361) -> ("Angle"=w303:dbl)  [unwired: 7 in, 3 out]
        n158 = call <vilib>:"WPI_EncoderGet.vi"("EncoderDevRef"=w360) -> ("Distance"=w342:dbl, "EncoderDevRef"=w353:T30, "Rate"=w312:dbl)  [unwired: 5 in, 3 out]
        n159 = Wait (ms)(milliseconds to wait=u32 20) -> ()  [unwired: 1 out]
        n160 = call "Gyro_Continuous.vi"("GyroInitial"=w303, "GyroInput"=w303) -> ("GyroContinuous"=w355:dbl)  [unwired: 9 in]
        n161 = call "FILTER_BOX_10.vi"("Input"=w303) -> ()  [unwired: 10 in, 1 out]
        n162 = call "FILTER_BOX_10.vi"("Input"=w312) -> ()  [unwired: 10 in, 1 out]
        n163 = call "FILTER_BOX_10.vi"("Input"=w313) -> ()  [unwired: 10 in, 1 out]
        n164 = call "Integrate.vi"("Elapsed Sec"=w320, "Rate"=w312) -> ("DIST"=w318:dbl)  [unwired: 9 in]
        n165 = call "Integrate.vi"("Elapsed Sec"=w320, "Rate"=w313) -> ("DIST"=w319:dbl)  [unwired: 9 in]
        n166 = call "TIME_GET.vi"() -> ("TIME"=w309:dbl)  [unwired: 10 in, 1 out]
        n167 = case shown="\"Autonomous Enabled\"" w366 {
          tunnel: w348 -> [_ w386]
          tunnel: [0 w385] -> w364
          tunnel: w361 -> [w372 _]
          tunnel: w355 -> [_ w384]
          tunnel: [w368 w383] -> w354
          tunnel: w359 -> [w371 _]
          tunnel: w318 -> [_ w382]
          tunnel: "Enable Ramsete" -> [_ w381]
          tunnel: w353 -> [w370 _]
          tunnel: w350 -> [_ w380]
          tunnel: w349 -> [_ w378]
          tunnel: [w368 w377] -> w310
          tunnel: [w368 w376] -> w308
          tunnel: w319 -> [_ w375]
          tunnel: w305 -> [_ w374]
          tunnel: w309 -> [_ w373]
          frame "Autonomous Disabled", Default {
            w368 = 0.0
            n168 = call <vilib>:"WPI_EncoderReset.vi"("EncoderDevRef"=w370) -> ()  [unwired: 9 in, 2 out]
            n169 = call <vilib>:"WPI_EncoderReset.vi"("EncoderDevRef"=w371) -> ()  [unwired: 9 in, 2 out]
            n170 = call <vilib>:"WPI_GyroReset.vi"("GyroDevRef"=w372) -> ()  [unwired: 9 in, 2 out]
          }
          frame "Autonomous Enabled" {
            # "Dist"
            n171 = case shown="True" TRUE {
              tunnel: w386 -> [w389 w391]
              tunnel: [w389 w424] -> w385
              tunnel: w384 -> [w388 w413]
              tunnel: [w388 w413] -> w383
              tunnel: w382 -> [_ w420]
              tunnel: w375 -> [_ w418]
              tunnel: w381 -> [_ w419]
              tunnel: w380 -> [_ w421]
              tunnel: w378 -> [_ w404]
              tunnel: [w387 w407] -> w377
              tunnel: [w387 w406] -> w376
              tunnel: w374 -> [_ w402]
              tunnel: w373 -> [_ w394]
              frame False {
                w387 = 0.0
              }
              frame True {
                # "ensure speed <=\nmax"
                # "try look ahead...."
                # "run ramsette"
                n172 = Equal To 0?(x=w391) -> (x = 0?=w399:bool)
                n173 = Increment(x=w391) -> (x+1=w424:i32)
                n174 = feedback #6() -> (w414:dbl)  [unwired: 1 in]
                n175 = case shown="False" w399 {
                  tunnel: w394 -> [_ w426]
                  tunnel: [w425 w426] -> w415
                  tunnel: w414 -> [w425 _]
                  frame False {
                  }
                  frame True {
                  }
                }
                n176 = Subtract(x=w394, y=w415) -> (x-y=w412:dbl)
                n177 = feedback-in #6(w415) -> ()
                n178 = Multiply(x=50.0, y=w412) -> (x*y=w410:dbl)
                n179 = To Long Integer(number=w410) -> (32bit integer=w390:i32)
                n180 = Max & Min(x=w404, y=w390) -> (min(x,y)=w400:i32)  [unwired: 1 out]
                n181 = Add(x=0, y=w400) -> (x+y=w403:i32)
                n182 = Max & Min(x=w403, y=w404) -> (min(x,y)=w401:i32)  [unwired: 1 out]
                n183 = Index Array(array=w421, index #1=w400, index #2=w401) -> (element #1=w392:T8, element #2=w398:T8)
                "element" <- w392
                n184 = Unbundle By Name(w398) -> ("Path X"=w397:dbl, "Path Y"=w396:dbl, "Path Heading"=w395:dbl)
                n185 = Bundle By Name(cluster=w392, "Path X"=w397, "Path Y"=w396, "Path Heading"=w395) -> ()  [unwired: 1 out]
                n186 = call "Do_Ramsete_Eng.vi"("LeftDist-Feet"=w420, "WheelBase-Feet"=1.738, "RightDist-Feet"=w418, "Ramsete Enable"=w419, "Path Sample"=w392, "Reset"=w399, "Gyro-Deg"=w413) -> ("AtReference"=→"AtReference":bool, "RightVelDmd"=w408:dbl, "LeftVelDmd"=w409:dbl, "CurrentRelativePose"=→"CurrentRelativePose":T9, "Err Pose"=→"Err Pose":T9)
                n187 = call "Wheel_Normalize.vi"("Max Speed"=w402, "Right Wheel Demand"=w408, "Left Wheel Demand"=w409) -> ("Normalized Right Wheel Demand"=w406:dbl, "Normalized Left Wheel Demand"=w407:dbl)  [unwired: 7 in]
                n188 = call "Path_To_Pose_Eng.vi"("Path Sample"=w392) -> ("out POSe"=→"Des Pose":T9)  [unwired: 10 in]
              }
            }
          }
        }
        "Heading" <- w354
        n189 = Multiply(x=w343, y=w342) -> (x*y=w340:dbl)
        n190 = Multiply(x=w343, y=w321) -> (x*y=w341:dbl)
        n191 = Multiply(x=2.5, y=w305) -> (x*y=w304:dbl)
        n192 = call "RATE_LIMIT.vi"("Max Rate"=w304, "Input"=w308) -> ("Limited Output"=w307:dbl)  [unwired: 9 in]
        n193 = call "RATE_LIMIT.vi"("Max Rate"=w304, "Input"=w310) -> ("Limited Output"=w311:dbl)  [unwired: 9 in]
        n194 = Multiply(x=w307, y=w322) -> (x*y=w324:dbl)
        n195 = Multiply(x=w311, y=w322) -> (x*y=w323:dbl)
        n196 = Multiply(x=w313, y=w322) -> (x*y=w330:dbl)
        n197 = Multiply(x=w312, y=w322) -> (x*y=w325:dbl)
        n198 = Replace Array Subset(array=w337, new element #1=w312, new element #2=w313) -> (w346:dbl[])  [unwired: 2 in]
        "Speed" <- w346
        n199 = call-poly <vilib>:"PID.vi"("output range"=w329, "PID gains"="Speed PID", "process variable"=w325, "setpoint"=w323) -> ("output"=w336:dbl)  [unwired: 6 in, 1 out]
        n200 = call-poly <vilib>:"PID.vi"("output range"=w329, "PID gains"="Speed PID", "process variable"=w330, "setpoint"=w324) -> ("output"=w334:dbl)  [unwired: 6 in, 1 out]
        n201 = Replace Array Subset(array=w339, new element #1=w318, new element #2=w319) -> (w356:dbl[])  [unwired: 2 in]
        "Distance" <- w356
        n202 = Replace Array Subset(array=w338, new element #1=w340, new element #2=w341) -> (w344:dbl[])  [unwired: 2 in]
        "DistRead" <- w344
        n203 = call-poly <vilib>:"NT Write Value.vi"("Numeric"=w354, "Name"="Gyro") -> ()  [unwired: 9 in, 1 out]
        n204 = Add(x=w334, y=w324) -> (x+y=w333:dbl)
        n205 = Add(x=w336, y=w323) -> (x+y=w335:dbl)
        n206 = call-poly <vilib>:"NT Write Value.vi"("Numeric Array"=w346, "Name"="Drive/Speed") -> ()  [unwired: 9 in, 1 out]
        n207 = call-poly <vilib>:"NT Write Value.vi"("Numeric Array"=w356, "Name"="Drive/Distance") -> ()  [unwired: 9 in, 1 out]
        n208 = In Range and Coerce(upper limit=w331, x=w333, lower limit=w332) -> (coerced(x)=w326:dbl)  [unwired: 1 out]
        n209 = In Range and Coerce(upper limit=w331, x=w335, lower limit=w332) -> (coerced(x)=w327:dbl)  [unwired: 1 out]
        n210 = call-poly <vilib>:"NT Write Value.vi"("Numeric Array"=w344, "Name"="Drive/DistanceRead") -> ()  [unwired: 9 in, 1 out]
        n211 = call <vilib>:"WPI_RobotDriveMotors.vi"("RightSpeed"=w326, "LeftSpeed"=w327, "RobotDriveDevRef"=w365) -> ("Motor Values"=w314:dbl[])  [unwired: 6 in, 2 out]
        "MotorOut" <- w314
        n212 = Replace Array Subset(array=w315, new element #1=w311, new element #2=w307) -> (w316:dbl[])  [unwired: 2 in]
        "SpeedDmd" <- w316
        n213 = call-poly <vilib>:"NT Write Value.vi"("Numeric Array"=w314, "Name"="DriveMotors") -> ()  [unwired: 9 in, 1 out]
        n214 = call-poly <vilib>:"NT Write Value.vi"("Numeric Array"=w316, "Name"="Drive/SpeedDmd") -> ()  [unwired: 9 in, 1 out]
        "Path INX" <- w348
      }
      n215 = while {
        stop <- FALSE stop-if-true
        n216 = case shown="True" "Stop\nProgram" {
          frame False {
          }
          frame True {
            n217 = Stop() -> ()  [unwired: 1 in]
          }
        }
        n218 = Wait (ms)(milliseconds to wait=u32 100) -> ()  [unwired: 1 out]
      }
      "Robot\nExecuting" <- TRUE ("Robot\nExecuting")
    }
  }
